vi "Update Plugin Address Control.vi"(8 "error in (no error)":errorcluster, 10 "Loaded Plugins":refnum<vi>, 11 "IP":string) -> (0 "error out":errorcluster, 3 "Plugin Address":string)   [LabVIEW 2021, in "CIF_UI.lvclass"]
uses:
  CIF_UI.lvclass
  CIF_UI.lvclass/CIF_UI.ctl
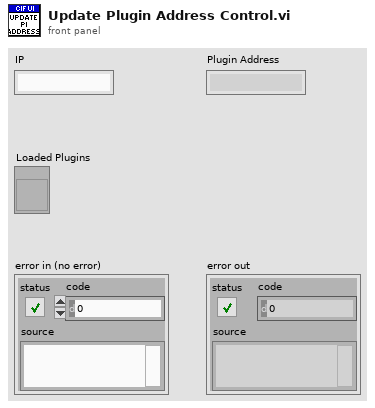
[diagram p1: front panel]
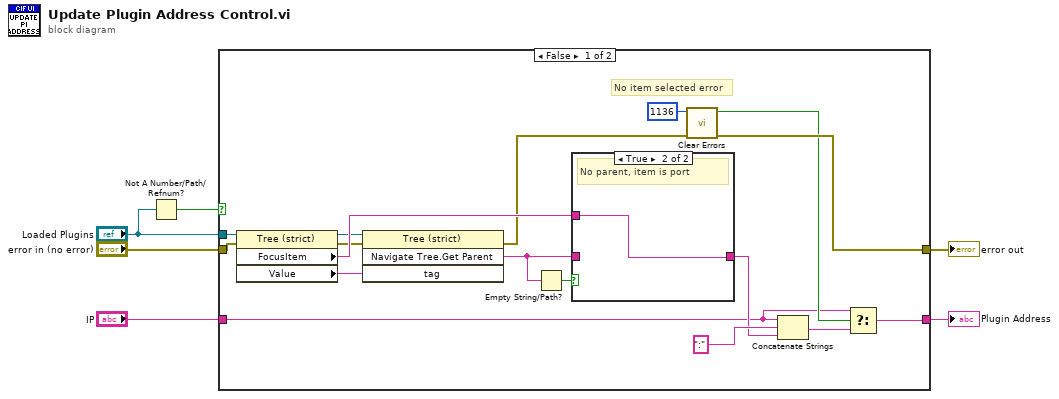
[diagram p0: block diagram]
diagram:
  n1 = Not A Number/Path/Refnum?(number/path/refnum="Loaded Plugins") -> (NaN/Path/Refnum?=w1:bool)
  n2 = case shown="False" w1 {
    tunnel: "error in (no error)" -> [w17 w26]
    tunnel: "IP" -> [w7 w25]
    tunnel: [w12 w26] -> w4
    tunnel: [w10 w25] -> w3
    tunnel: "Loaded Plugins" -> [w8 _]
    frame False {
      # "No item selected error"
      n3 = property class="Tree (strict)"(reference=w8, error in=w17) -> (error out=w18:errorcluster, "FocusItem"=w19:string, "Value"=w22:string)  [unwired: 1 out]
      n4 = invoke class="Tree (strict)" method="Navigate Tree.Get Parent"(reference=w8, error in=w18, "tag"=w22) -> (error out=w13:errorcluster, "Navigate Tree:Get Parent"=w20:string)  [unwired: 1 in, 2 out]
      n5 = Empty String/Path?(string/path=w20) -> (empty?=w21:bool)
      n6 = case shown="True" w21 {
        tunnel: w20 -> [w23 _]
        tunnel: w19 -> [_ w24]
        tunnel: [w23 w24] -> w15
        frame False {
          # "Parent is port"
        }
        frame True {
          # "No parent, item is port"
        }
      }
      n7 = call <vilib>:"Clear Errors.vi"("error in (no error)"=w13, "specific error code to clear (0: all)"=1136) -> ("error out"=w12:errorcluster, "specific error cleared?"=w9:bool)  [unwired: 4 in]
      n8 = Concatenate Strings(w7, ":" ("string"), w15) -> (w11:string)
      n9 = Select(t=w7, s=w9, f=w11) -> (s? t:f=w10:string)
    }
    frame True {
    }
  }
  "error out" <- w4
  "Plugin Address" <- w3
